vi "GNSS1-set-1.vi"(0 "gps收星数":refnum<vi>, 1 "GPS故障字低4位":refnum<vi>, 3 "GPS定位状态":refnum<vi>, 5 "gps-pdop":refnum<vi>, 7 "spare":refnum<vi>, 9 "GPS故障字高4位":refnum<vi>, 11 "gps时间差":refnum<vi>, 12 "gps北京时间":refnum<vi>, 13 "gps速度位置":refnum<vi>) -> (4 "添加的数组1":u8[](array[numeric]))   [LabVIEW 2012]
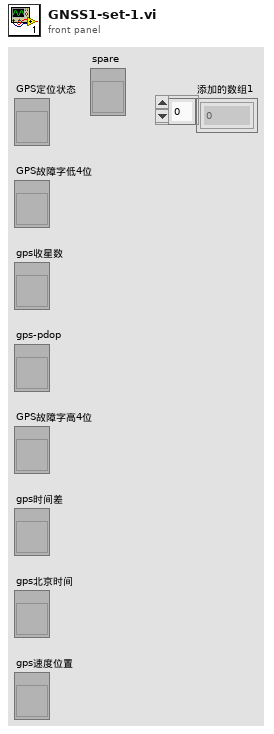
[diagram p1: front panel]
types:
  T1 = typedef "LVDateTimeRec.ctl" = cluster{"秒数的小数部分":dbl, "秒":i32, "分":i32, "时":i32, "日":i32, "月":i32, "年":i32, "天数（周）":i32, "天数（年）":i32, "DST":i32}
  T2 = cluster{"GPS北向速度":sgl, "GPS东向速度":sgl, "GPS地向速度":sgl, "GPS经度":sgl, "GPS纬度":sgl, "GPS高度":sgl}
  T3 = enum8{"无故障", "未正常初始化", "PDOP值>12", "没有可用卫星", "只有1颗可用卫星", "只有2颗可用卫星", "只有3颗可用卫星", "观测矩阵不可求逆", "定位解算不收敛", "高程超差", "速度大于10km/s"}
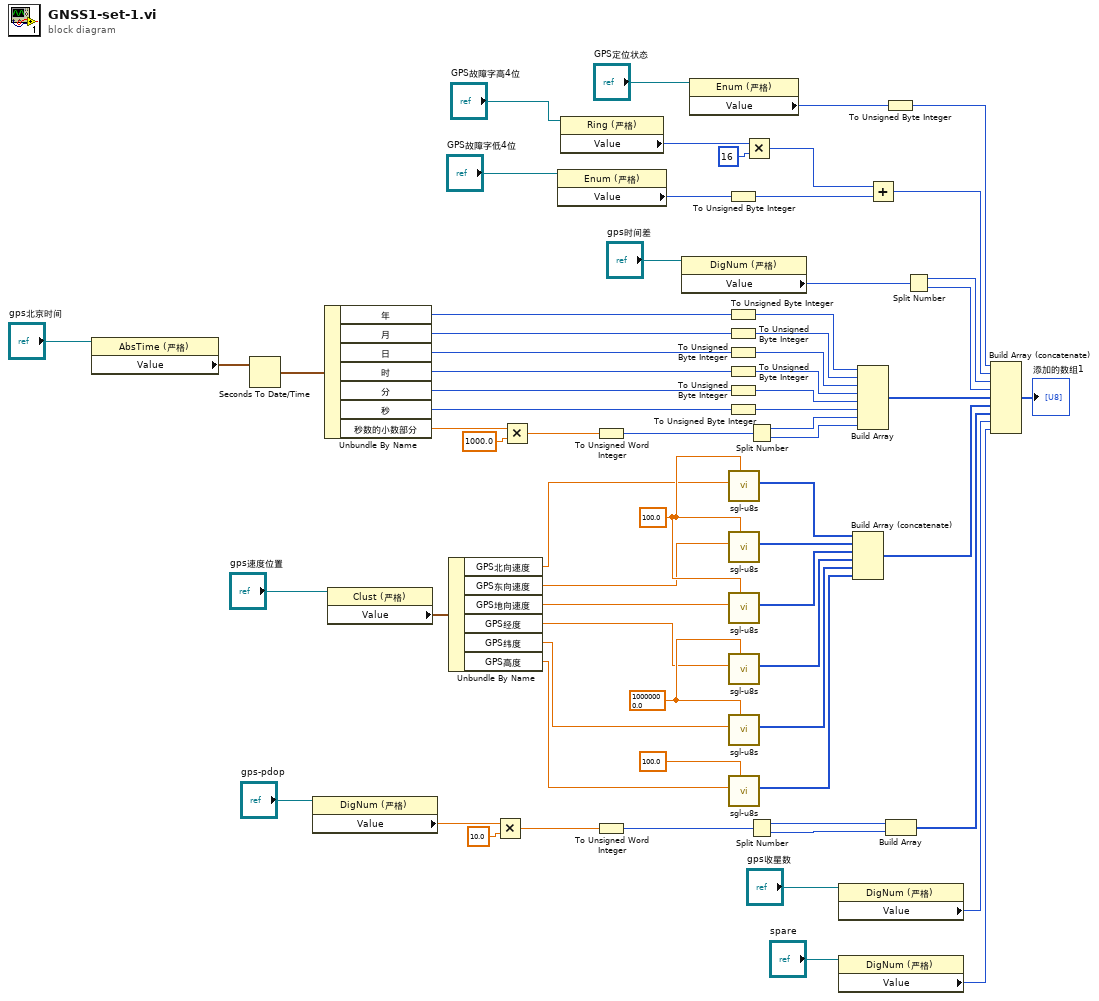
[diagram p0: block diagram]
diagram:
  w66 = sgl 10000000.0 ("精度")
  w48 = sgl 100.0 ("y")
  n1 = property on="属性节点" class="AbsTime (严格)"(reference="gps北京时间") -> ("Value"=w39:timestamp)  [unwired: 1 in, 2 out]
  n2 = Seconds To Date/Time(time stamp (now)=w39) -> (date time rec=w20:T1)  [unwired: 1 in]
  n3 = property on="属性节点" class="DigNum (严格)"(reference="gps-pdop") -> ("Value"=w61:sgl)  [unwired: 1 in, 2 out]
  n4 = Unbundle By Name(w20) -> ("年"=w21:i32, "月"=w23:i32, "日"=w24:i32, "时"=w25:i32, "分"=w26:i32, "秒"=w27:i32, "秒数的小数部分"=w28:dbl)
  n5 = property on="属性节点" class="Clust (严格)"(reference="gps速度位置") -> ("Value"=w54:T2)  [unwired: 1 in, 2 out]
  n6 = Unbundle By Name(w54) -> ("GPS北向速度"=w41:sgl, "GPS东向速度"=w43:sgl, "GPS地向速度"=w44:sgl, "GPS经度"=w45:sgl, "GPS纬度"=w46:sgl, "GPS高度"=w47:sgl)
  n7 = Multiply(x=w61, y=sgl 10.0) -> (x*y=w57:sgl)
  n8 = Multiply(x=w28, y=1000.0) -> (x*y=w30:dbl)
  n9 = property on="属性节点" class="Enum (严格)"(reference="GPS故障字低4位") -> ("Value"=w14:T3)  [unwired: 1 in, 2 out]
  n10 = property on="属性节点" class="Ring (严格)"(reference="GPS故障字高4位") -> ("Value"=w11:u8)  [unwired: 1 in, 2 out]
  n11 = To Unsigned Word Integer(number=w30) -> (unsigned 16bit integer=w31:u16)
  n12 = To Unsigned Word Integer(number=w57) -> (unsigned 16bit integer=w60:u16)
  n13 = property on="属性节点" class="DigNum (严格)"(reference="gps时间差") -> ("Value"=w17:u16)  [unwired: 1 in, 2 out]
  n14 = property on="属性节点" class="Enum (严格)"(reference="GPS定位状态") -> ("Value"=w64:enum8{"无效", "定点定位", "差分定位"})  [unwired: 1 in, 2 out]
  n15 = To Unsigned Byte Integer(number=w14) -> (unsigned 8bit integer=w15:u8)
  n16 = To Unsigned Byte Integer(number=w21) -> (unsigned 8bit integer=w22:u8)
  n17 = To Unsigned Byte Integer(number=w23) -> (unsigned 8bit integer=w32:u8)
  n18 = To Unsigned Byte Integer(number=w24) -> (unsigned 8bit integer=w33:u8)
  n19 = To Unsigned Byte Integer(number=w25) -> (unsigned 8bit integer=w34:u8)
  n20 = To Unsigned Byte Integer(number=w26) -> (unsigned 8bit integer=w35:u8)
  n21 = To Unsigned Byte Integer(number=w27) -> (unsigned 8bit integer=w36:u8)
  n22 = call "sgl-u8s.vi"("输入sgl"=w41, "精度"=w48) -> ("u8s"=w42:u8[])  [unwired: 8 in]
  n23 = call "sgl-u8s.vi"("输入sgl"=w43, "精度"=w48) -> ("u8s"=w49:u8[])  [unwired: 8 in]
  n24 = call "sgl-u8s.vi"("输入sgl"=w44, "精度"=w48) -> ("u8s"=w50:u8[])  [unwired: 8 in]
  n25 = call "sgl-u8s.vi"("输入sgl"=w45, "精度"=w66) -> ("u8s"=w51:u8[])  [unwired: 8 in]
  n26 = call "sgl-u8s.vi"("输入sgl"=w46, "精度"=w66) -> ("u8s"=w52:u8[])  [unwired: 8 in]
  n27 = call "sgl-u8s.vi"("输入sgl"=w47, "精度"=sgl 100.0) -> ("u8s"=w53:u8[])  [unwired: 8 in]
  n28 = Multiply(x=w11, y=u8 16) -> (x*y=w13:u8)
  n29 = Split Number(x=w31) -> (hi(x)=w37:u8, lo(x)=w38:u8)
  n30 = Split Number(x=w60) -> (hi(x)=w58:u8, lo(x)=w59:u8)
  n31 = property on="属性节点" class="DigNum (严格)"(reference="gps收星数") -> ("Value"=w63:u8)  [unwired: 1 in, 2 out]
  n32 = property on="属性节点" class="DigNum (严格)"(reference="spare") -> ("Value"=w2:u8)  [unwired: 1 in, 2 out]
  n33 = Build Array (concatenate)(w42, w49, w50, w51, w52, w53) -> (w55:u8[])
  n34 = Build Array(w22, w32, w33, w34, w35, w36, w37, w38) -> (w40:u8[])
  n35 = Add(x=w13, y=w15) -> (x+y=w16:u8)
  n36 = To Unsigned Byte Integer(number=w64) -> (unsigned 8bit integer=w65:u8)
  n37 = Build Array(w58, w59) -> (w62:u8[])
  n38 = Split Number(x=w17) -> (hi(x)=w18:u8, lo(x)=w19:u8)
  n39 = Build Array (concatenate)(w65, w16, w18, w19, w40, w55, w62, w63, w2) -> (→"添加的数组1":u8[])
